vi "Rotate Lidar Data.vi"(10 "Angle (rad)":dbl, 11 "Raw Lidar Data":cluster{dbl[], dbl[]}(graph)={array[569 elements], array[569 elements]}) -> (3 "Rotated Lidar Data":cluster{dbl[], dbl[]}(graph))   [LabVIEW 2017]
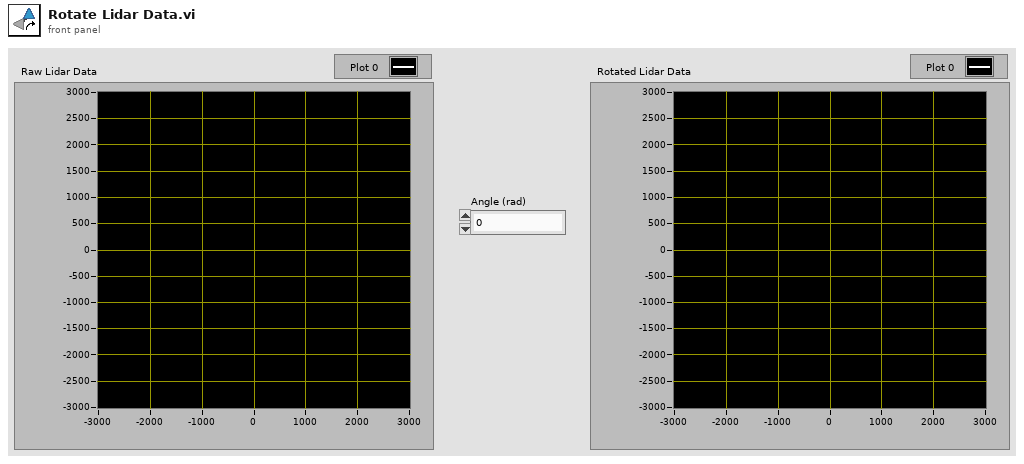
[diagram p1: front panel]
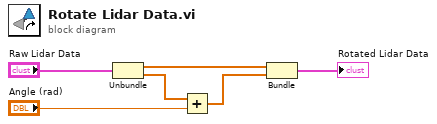
[diagram p0: block diagram]
diagram:
  n1 = Unbundle("Raw Lidar Data") -> (w2:dbl[], w4:dbl[])
  n2 = Add(x=w4, y="Angle (rad)") -> (x+y=w3:dbl[])
  n3 = Bundle(w2, w3) -> (→"Rotated Lidar Data":cluster{dbl[], dbl[]})  [unwired: 1 in]
